vi "Run Test- Data view (eFGV).vi"(7 "eFGV States":T1, 8 "error in (no error)":errorcluster, 11 "Data view in":bool) -> (0 "error out":errorcluster, 2 "Data view":refnum<user-event>, 3 "Data view out":bool)   [LabVIEW 2019]
uses:
  Controls/eFGV States.ctl
  <vilib>/event_ctls.llb/usereventprio.ctl
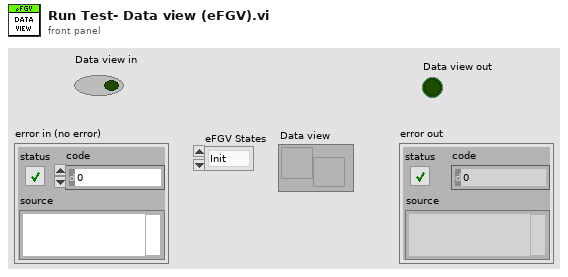
[diagram p1: front panel]
types:
  T1 = typedef "eFGV States.ctl" = enum16{"Init", "Read", "Write", "Exit"}
  T2 = typedef "usereventprio.ctl" = enum32{"high priority", "normal priority"}
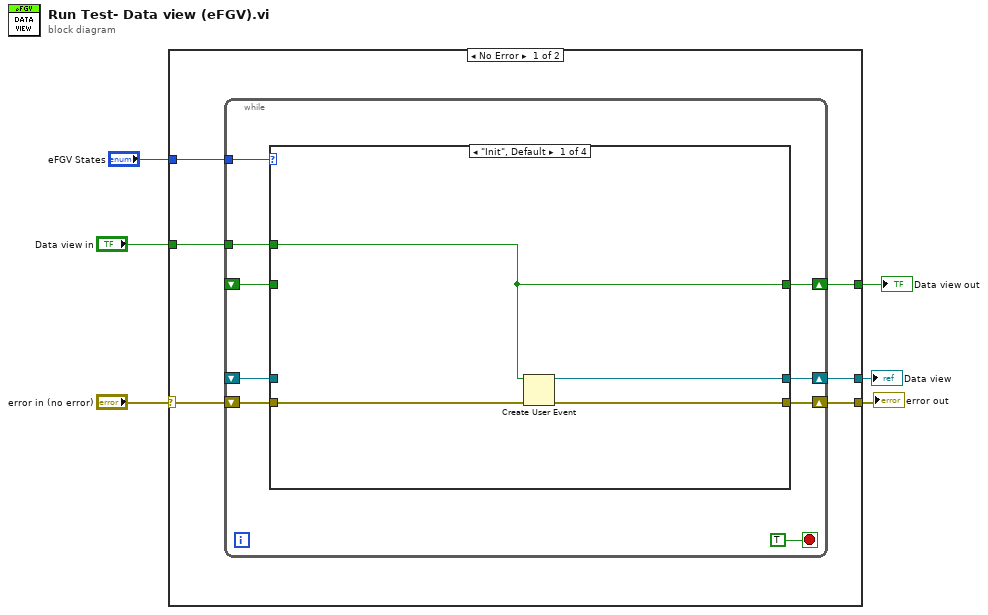
[diagram p0: block diagram]
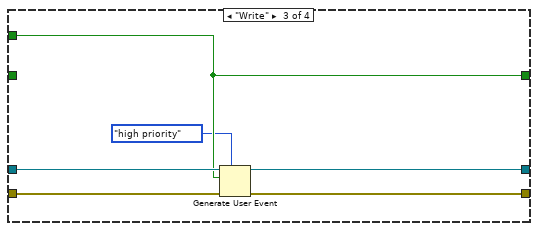
[diagram p3: hidden frame]
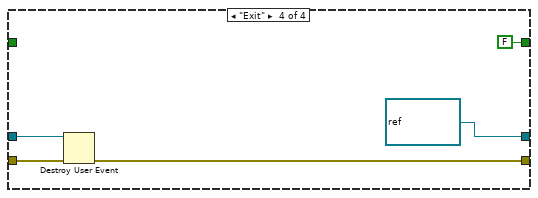
[diagram p4: hidden frame]
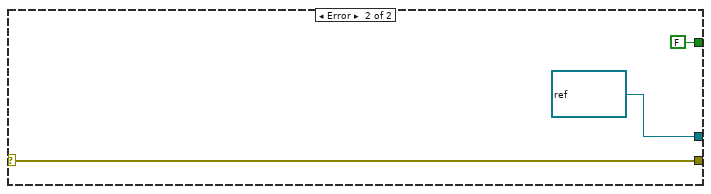
[diagram p5: hidden frame]
diagram:
  n1 = case shown="No Error" "error in (no error)" {
    selector: "error in (no error)" -> [w11 w40]
    tunnel: "eFGV States" -> [w12 _]
    tunnel: "Data view in" -> [w10 _]
    tunnel: [w9 w40] -> w2
    tunnel: [w8 refnum<user-event> refnum ("Exit In")] -> w3
    tunnel: [w7 FALSE ("Exit In")] -> w1
    frame No Error {
      n2 = while {
        tunnel: w12 -> [w20]
        shift-right: [w17] -> w9
        shift-left: w11 -> [w19]
        tunnel: w10 -> [w18]
        shift-right: [w16] -> w7
        shift-left: _ -> [w15]
        shift-right: [w14] -> w8
        shift-left: _ -> [w13]
        stop <- TRUE stop-if-true
        n3 = case shown="\"Init\", Default" w20 {
          tunnel: w19 -> [w25 w26 w31 w39]
          tunnel: w18 -> [w23 _ w30 _]
          tunnel: [w24 w26 w32 w37] -> w17
          tunnel: [w23 w28 w30 FALSE ("Exit In")] -> w16
          tunnel: w15 -> [_ w28 _ _]
          tunnel: [w22 w27 w33 refnum<user-event> refnum ("Exit In")] -> w14
          tunnel: w13 -> [_ w27 w34 w38]
          frame "Init", Default {
            n4 = Create User Event(user event datatype=w23, error in=w25) -> (user event=w22:refnum<user-event>, error out=w24:errorcluster)
          }
          frame "Read" {
          }
          frame "Write" {
            n5 = Generate User Event(priority (normal)=usereventprio."high priority", user event=w34, event data cluster=w30, error in=w31) -> (user event out=w33:refnum<user-event>, error out=w32:errorcluster)
          }
          frame "Exit" {
            n6 = Destroy User Event(user event=w38, error in=w39) -> (error out=w37:errorcluster)
          }
        }
      }
    }
    frame Error {
    }
  }
  "error out" <- w2
  "Data view out" <- w1
  "Data view" <- w3
